vi "Check Left Right Button.vi"(8 "error in (no error)":errorcluster) -> (0 "error out":errorcluster, 1 "Right":bool, 2 "Left":bool, 3 "MouseButton":T1)   [LabVIEW 2021]
uses:
  <vilib>/Utility/inputDevices.llb/mouseAcquire.vi
  <vilib>/Utility/inputDevices.llb/closeMouse.vi
  <userlib>/John_Lib/Mouse/MouseButton.ctl
panel:
  out "Bolean String":string
  out "button info":T2
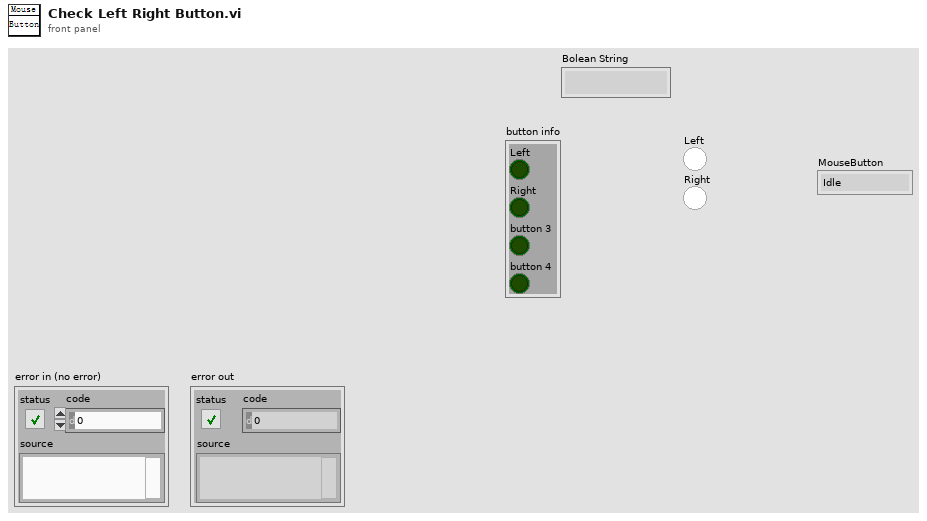
[diagram p1: front panel]
types:
  T1 = typedef "MouseButton.ctl" = enum16{"Idle", "Left", "Right", "Middle"}
  T2 = cluster{"Left":bool, "Right":bool, "button 3":bool, "button 4":bool}
  T3 = cluster{"button 1":bool, "button 2":bool, "button 3":bool, "button 4":bool}
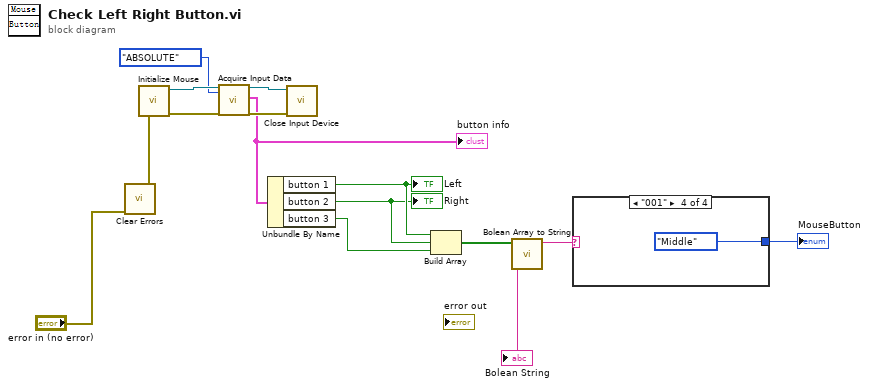
[diagram p0: block diagram]
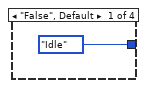
[diagram p2: hidden frame]
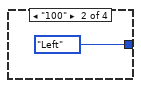
[diagram p3: hidden frame]
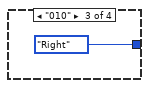
[diagram p4: hidden frame]
diagram:
  n1 = call <vilib>:"Clear Errors.vi"("error in (no error)"="error in (no error)") -> ("error out"=w11:errorcluster)  [unwired: 5 in, 1 out]
  n2 = call <vilib>:"Initialize Mouse.vi"("error in (no error)"=w11) -> ("error out"=w13:errorcluster, "device ID"=w14:refnum<k1>)  [unwired: 9 in]
  n3 = call-poly <vilib>:"Acquire Input Data.vi"("device ID"=w14, "key mode"=enum16{"RELATIVE", "ABSOLUTE"}."ABSOLUTE", "error in (no error)"=w13) -> ("device ID"=w8:refnum<k1>, "button info"=w7:T3, "error out"=w10:errorcluster)  [unwired: 13 in, 1 out]
  "button info" <- w7
  n4 = Unbundle By Name(w7) -> ("button 1"=w5:bool, "button 2"=w4:bool, "button 3"=w3:bool)
  "Right" <- w4
  "Left" <- w5
  n5 = call-poly <vilib>:"Close Input Device.vi"("error in (no error)"=w10, "device ID"=w8) -> ()  [unwired: 8 in, 1 out]
  n6 = Build Array(w5, w4, w3) -> (w2:bool[])
  n7 = call <userlib>:"Bolean Array to String.vi"("Bolean Array"=w2) -> ("Bolean String"=w6:string)  [unwired: 10 in]
  "Bolean String" <- w6
  n8 = case shown="\"001\"" w6 {
    tunnel: [MouseButton."Idle" ("MouseButton") MouseButton."Left" ("MouseButton") MouseButton."Right" ("MouseButton") MouseButton."Middle" ("MouseButton")] -> w1
    frame "False", Default {
    }
    frame "100" {
    }
    frame "010" {
    }
    frame "001" {
    }
  }
  "MouseButton" <- w1
